vi "generador_reporte_post_portada_subvi.vi"(11 "Array 2":cluster{"Class":string, string, string}[](array[cluster])) -> ()   [LabVIEW 2021]
uses:
  <vilib>/Utility/NIReport.llb/Report Type.ctl
  <vilib>/Utility/NIReport.llb/Append Report Text (str wrap).vi
  <vilib>/Utility/NIReport.llb/Append Image to Report (path wrap).vi
  <vilib>/Utility/NIReport.llb/NI_report.lvclass
  <vilib>/Utility/NIReport.llb/NI_ReportGenerationCore.lvlib
panel:
  out "appended path":path
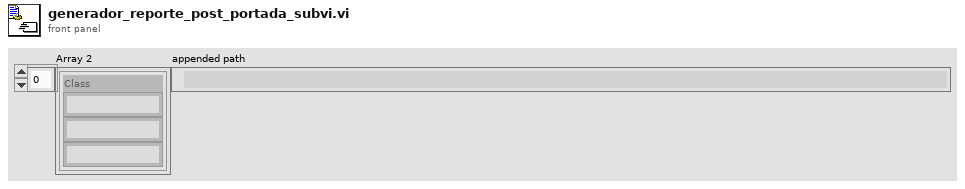
[diagram p1: front panel]
types:
  T1 = cluster{"Charset (-1)":i16, "Weight (-1)":i16, "Name":string, "Size":string}
  T2 = cluster{"Italic":enum16{"Italic Unchanged", "Italic On", "Italic Off"}, "Strike Through":enum16{"Strike Through Unchanged", "Strike Through On", "Strike Through Off"}, "Underline":enum16{"Underline Unchanged", "Underline On", "Underline Off"}, "Bold":enum16{"Bold Unchanged", "Bold On", "Bold Off"}}
  T3 = typedef "NI_ReportGenerationCore.lvlib/Report Type.ctl" = enum16{"HTML", "Word", "Excel"}
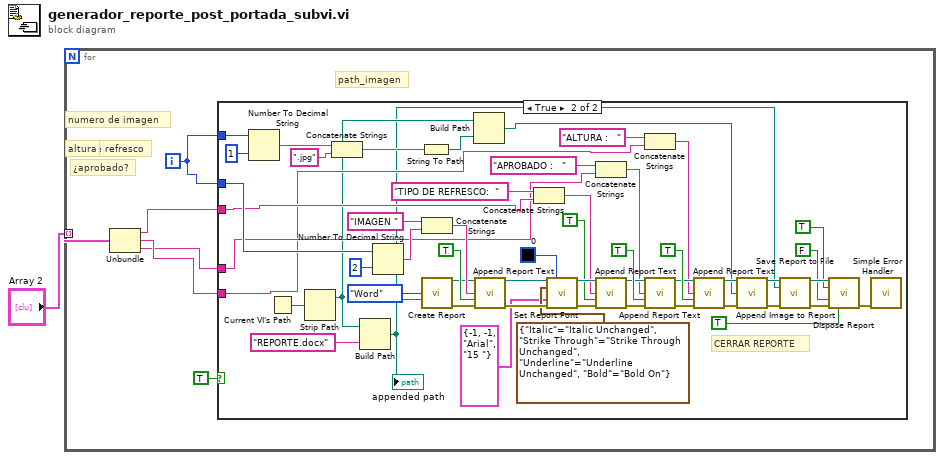
[diagram p0: block diagram]
diagram:
  n1 = for {
    tunnel: "Array 2" -> [w6] mode=indexing
    i -> [w5]
    # "path_imagen"
    # "altura"
    # "¿aprobado?"
    # "tipo de refresco"
    # "numero de imagen"
    n2 = Unbundle(w6) -> ("Class"=w4:string, w3:string, w2:string)
    n3 = case shown="True" TRUE {
      tunnel: w5 -> [_ w48]
      tunnel: w4 -> [_ w41]
      tunnel: w2 -> [_ w38]
      tunnel: w5 -> [_ w15]
      tunnel: w3 -> [_ w12]
      frame False {
      }
      frame True {
        # "CERRAR REPORTE"
        n4 = Number To Decimal String(number=w15, width (-)=i16 1) -> (decimal integer string=w18:string)
        n5 = Current VI's Path() -> (path=w21:path)
        n6 = Strip Path(path=w21) -> (stripped path=w10:path)  [unwired: 1 out]
        n7 = Concatenate Strings(w18, ".jpg" ("string")) -> (w19:string)
        n8 = Build Path(base path=w10, name or relative path="REPORTE.docx") -> (appended path=w8:path)
        "appended path" <- w8
        n9 = Number To Decimal String(number=w48, width (-)=i16 2) -> (decimal integer string=w47:string)
        n10 = String To Path(string=w19) -> (path=w20:path)
        n11 = Concatenate Strings("IMAGEN " ("text"), w47) -> (w46:string)
        n12 = call <vilib>:"Create Report.vi"("report type"=Report_Type."Word", "template (empty)"=w8) -> ("report out"=w14:refnum<class "NI_report.lvclass">, "error out"=w13:errorcluster)  [unwired: 12 in]
        n13 = Build Path(base path=w10, name or relative path=w20) -> (appended path=w11:path)
        n14 = call-poly <vilib>:"Append Report Text.vi"("report in"=w14, "text"=w46, "append on new line? (F)"=TRUE, "error in (no error)"=w13) -> ("report out"=w56:refnum<class "NI_report.lvclass">, "error out"=w55:errorcluster)  [unwired: 8 in, 2 out]
        n15 = Concatenate Strings("TIPO DE REFRESCO:  " ("text"), w41) -> (w40:string)
        n16 = call-dynamic "Set Report Font.vi"("report in"=w56, "text color (unchanged)"=u32 0, "text options"=T2 {"Italic"=enum."Italic Unchanged", "Strike Through"=enum."Strike Through Unchanged", "Underline"=enum."Underline Unchanged", "Bold"=enum."Bold On"}, "font settings"=T1 {"Charset (-1)"=-1, "Weight (-1)"=-1, "Name"="Arial", "Size"="15 "}, "error in (no error)"=w55) -> ("report out"=w45:refnum<class "NI_report.lvclass">, "error out"=w44:errorcluster)  [unwired: 8 in, 1 out]
        n17 = Concatenate Strings("APROBADO :   " ("text"), w38) -> (w30:string)
        n18 = call-poly <vilib>:"Append Report Text.vi"("report in"=w45, "text"=w40, "append on new line? (F)"=TRUE, "error in (no error)"=w44) -> ("report out"=w34:refnum<class "NI_report.lvclass">, "error out"=w31:errorcluster)  [unwired: 8 in, 2 out]
        n19 = Concatenate Strings("ALTURA :   " ("text"), w12) -> (w29:string)
        n20 = call-poly <vilib>:"Append Report Text.vi"("report in"=w34, "text"=w30, "append on new line? (F)"=TRUE, "error in (no error)"=w31) -> ("report out"=w33:refnum<class "NI_report.lvclass">, "error out"=w32:errorcluster)  [unwired: 8 in, 2 out]
        n21 = call-poly <vilib>:"Append Report Text.vi"("report in"=w33, "text"=w29, "append on new line? (F)"=TRUE, "error in (no error)"=w32) -> ("report out"=w25:refnum<class "NI_report.lvclass">, "error out"=w24:errorcluster)  [unwired: 8 in, 2 out]
        n22 = call-poly <vilib>:"Append Image to Report.vi"("report in"=w25, "path or URL of image"=w11, "error in (no error)"=w24) -> ("report out"=w22:refnum<class "NI_report.lvclass">, "error out"=w23:errorcluster)  [unwired: 9 in, 2 out]
        n23 = call-dynamic "Save Report to File.vi"("report in"=w22, "report file path"=w8, "error in (no error)"=w23) -> ("report out"=w60:refnum<class "NI_report.lvclass">, "error out"=w59:errorcluster)  [unwired: 11 in]
        n24 = call-dynamic "Dispose Report.vi"("report in"=w60, "wait until printing completed? (T)"=TRUE, "save changes? (F)"=FALSE, "error in (no error)"=w59, "close report? (T)"=TRUE) -> ("error out"=w51:errorcluster)  [unwired: 10 in]
        n25 = call <vilib>:"Simple Error Handler.vi"("error in (no error)"=w51) -> ()  [unwired: 4 in, 5 out]
      }
    }
  }
